vi "read_delay_time.vi"(8 "error in (no error)":errorcluster, 11 "config_file_name":string="config.ini") -> (0 "error out":errorcluster, 2 "values":cluster{"delay_time":string}, 3 "config_file_name_out":string)   [LabVIEW 2015]
uses:
  <vilib>/Utility/config.llb/Read Key (String).vi
  <vilib>/Utility/config.llb/NI_LVConfig.lvlib
panel:
  # "Devuelve datos de la sección DELAY TIME del archivo de configuración"
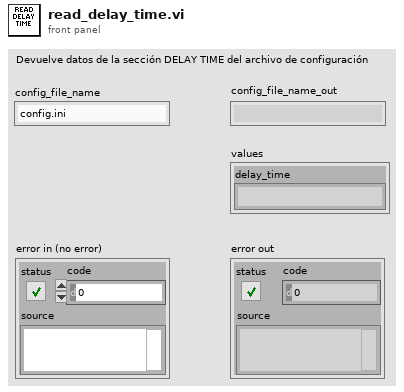
[diagram p1: front panel]
types:
  T1 = typedef "NI_LVConfig.lvlib/Config Data RefNum.ctl" = refnum<k1>
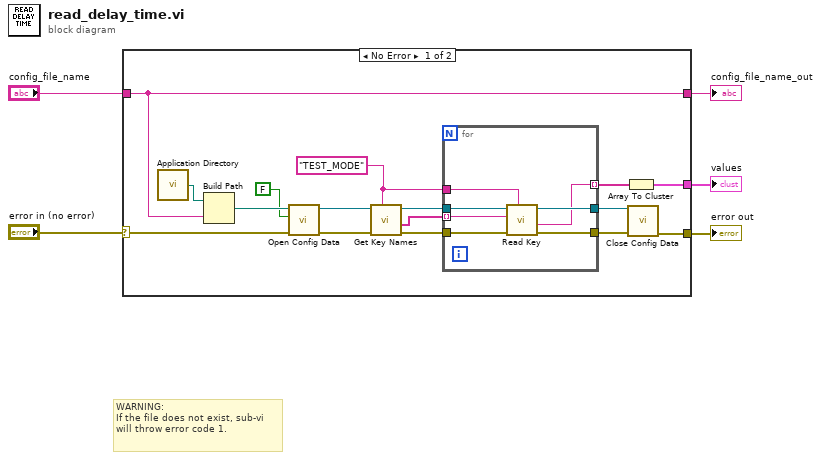
[diagram p0: block diagram]
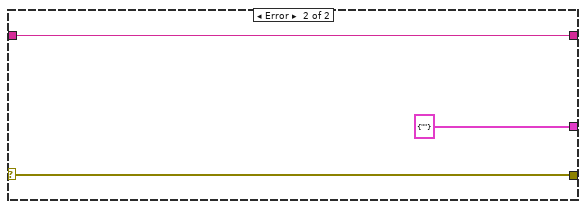
[diagram p2: hidden frame]
diagram:
  # "WARNING:\nIf the file does not exist, sub-vi will throw error code 1."
  n1 = case shown="No Error" "error in (no error)" {
    selector: "error in (no error)" -> [w11 w31]
    tunnel: [w10 w31] -> w5
    tunnel: [w7 cluster{"[0]":string} {"[0]"=""}] -> w3
    tunnel: "config_file_name" -> [w6 w30]
    tunnel: [w6 w30] -> w1
    frame No Error {
      w16 = "TEST_MODE" ("section")
      n2 = call <vilib>:"Application Directory.vi"() -> ("Application Directory"=w19:path)
      n3 = Build Path(base path=w19, name or relative path=w6) -> (appended path=w18:path)
      n4 = call <vilib>:"Open Config Data.vi"("error in (no error)"=w11, "create file if necessary (T)"=FALSE, "configuration file path"=w18) -> ("error out"=w21:errorcluster, "refnum"=w20:T1)  [unwired: 6 in, 1 out]
      n5 = call <vilib>:"Get Key Names.vi"("section"=w16, "error in (no error)"=w21, "refnum"=w20) -> ("error out"=w14:errorcluster, "key names"=w17:string[], "refnum out"=w15:T1)  [unwired: 5 in, 1 out]
      n6 = for {
        tunnel: w17 -> [w28] mode=indexing
        tunnel: [w22] -> w9 mode=indexing
        tunnel: w16 -> [w27]
        tunnel: w15 -> [w26]
        tunnel: w14 -> [w25]
        tunnel: [w24] -> w13
        tunnel: [w23] -> w12
        n7 = call-poly <vilib>:"Read Key.vi"("section"=w27, "error in (no error)"=w25, "key"=w28, "refnum"=w26) -> ("error out"=w23:errorcluster, "value"=w22:string, "refnum out"=w24:T1)  [unwired: 4 in, 1 out]
      }
      n8 = Array To Cluster(array=w9) -> (cluster=w7:cluster{"[0]":string})
      n9 = call <vilib>:"Close Config Data.vi"("error in (no error)"=w12, "refnum"=w13) -> ("error out"=w10:errorcluster)  [unwired: 8 in, 1 out]
    }
    frame Error {
    }
  }
  "error out" <- w5
  "values" <- w3
  "config_file_name_out" <- w1
